vi "Initialize Logging Data.vi"(8 "error in (no error)":errorcluster, 11 "Device Ref in":T2=18446744073709551615 format="%.0x") -> (0 "error out":errorcluster, 1 "File Sample Specs":T9[](array[typedef]) {"File Status Ref" format="%.0x"; "Cmd Ref" format="%.0x"; "Data Loss Ref" format="%.0x"; "Error Ref" format="%.0x"; "Groups"."Decimation Ref" format="%.0x"; "Groups"."Block Refs"."Data Reference" format="%.0x"; "Trigger Ref" format="%.0x"}, 2 "File Log Specs":T3[](array[typedef]) {"File Node Ref" format="%.0x"}, 3 "Device Ref out":T2=18446744073709551615 format="%.0x", 4 "Max Group Size":i32, 5 "FIFO % Ref":T1 format="%.0x", 6 "Max # Channel Groups":i32)   [LabVIEW 2027, in "Embedded Data Logger Engine.lvlib"]
uses:
  Embedded Data Logger Engine.lvlib
  File Sampling Specification.ctl
  <vilib>/NI VeriStand/Custom Device API/Data Reference.ctl
  Group Sampling Specification.ctl
  <vilib>/NI VeriStand/Custom Device API/Block Data Reference.ctl
  File Logging Specification.ctl
  Group Logging Specification.ctl
  Group Buffer Data.ctl
  Property Specification.ctl
  <vilib>/NI VeriStand/Custom Device API/Custom Device Item Ref.ctl
  Shared/Segment Files By.ctl
  Logging State.ctl
  <vilib>/NI VeriStand/Custom Device API/Data Access Type.ctl
  Shared/Constants.vi
  <vilib>/NI VeriStand/Custom Device Tools/Custom Device Utility Library/NI VeriStand - Search for All Items by GUID.vi
  <vilib>/NI VeriStand/Custom Device Tools/Custom Device Utility Library/NI VeriStand - Search for Item by GUID.vi
  <vilib>/NI VeriStand/Custom Device Tools/Custom Device Utility Library/NI VeriStand - Search for Item by Property.vi
  <vilib>/NI VeriStand/Custom Device API/Get Item Property (String Array).vi
  <vilib>/NI VeriStand/Custom Device Tools/Custom Device Utility Library/Custom Device Utility Library.lvlib
  <vilib>/NI VeriStand/Custom Device API/Custom Device API.lvlib
  Shared/Embedded Data Logger Shared.lvlib
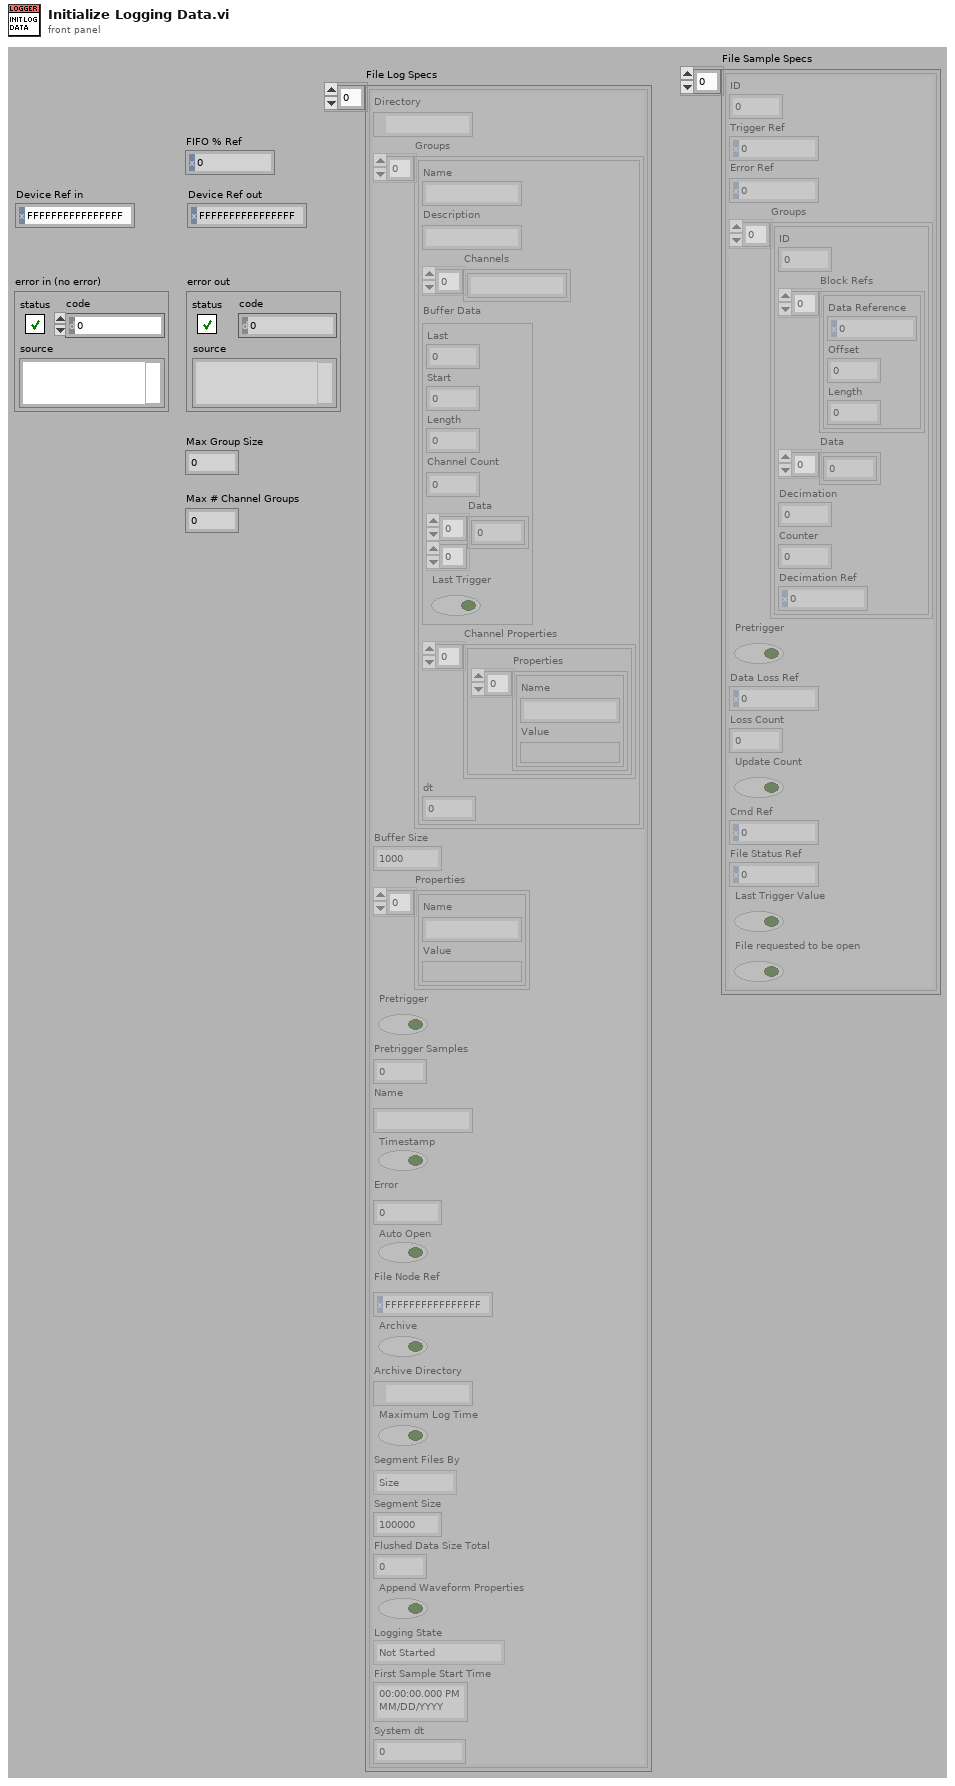
[diagram p1: front panel]
types:
  T1 = typedef "Custom Device API.lvlib/Data Reference.ctl" = i32
  T2 = typedef "Custom Device API.lvlib/Custom Device Item Ref.ctl" = u64
  T3 = typedef "Embedded Data Logger Engine.lvlib/File Logging Specification.ctl" = cluster{"Directory":path, "Groups":T4[], "Buffer Size":i32, "Properties":T6[], "Pretrigger":bool, "Pretrigger Samples":i32, "Name":string, "Timestamp":bool, "Error":i32, "Auto Open":bool, "File Node Ref":T2, "Archive":bool, "Archive Directory":path, "Segment Files":bool, "Segment Files By":T7, "Segment Size":u32, "Flushed Data Size Total":u32, "Append Waveform Properties":bool, "Logging State":T8, "First Sample Start Time":timestamp, "System dt":dbl}
  T4 = typedef "Embedded Data Logger Engine.lvlib/Group Logging Specification.ctl" = cluster{"Name":string, "Description":string, "Channels":string[], "Buffer Data":T5, "Channel Properties":cluster{"Properties":T6[]}[], "dt":dbl}
  T5 = typedef "Embedded Data Logger Engine.lvlib/Group Buffer Data.ctl" = cluster{"Last":i32, "Start":i32, "Length":i32, "Channel Count":i32, "Data":dbl[][], "Last Trigger":bool}
  T6 = typedef "Embedded Data Logger Engine.lvlib/Property Specification.ctl" = cluster{"Name":string, "Value":variant}
  T7 = typedef "Embedded Data Logger Shared.lvlib/Segment Files By.ctl" = enum16{"Time", "Size"}
  T8 = typedef "Embedded Data Logger Engine.lvlib/Logging State.ctl" = enum16{"Not Started", "Continous Logging", "Paused", "Discontinous Logging"}
  T9 = typedef "Embedded Data Logger Engine.lvlib/File Sampling Specification.ctl" = cluster{"ID":dbl, "Trigger Ref":T1, "Error Ref":T1, "Groups":T10[], "Pretrigger":bool, "Data Loss Ref":T1, "Loss Count":i32, "Update Count":bool, "Cmd Ref":T1, "File Status Ref":T1, "Last Trigger Value":bool, "File requested to be open":bool}
  T10 = typedef "Embedded Data Logger Engine.lvlib/Group Sampling Specification.ctl" = cluster{"ID":dbl, "Block Refs":T11[], "Data":dbl[], "Decimation":i32, "Counter":i32, "Decimation Ref":T1}
  T11 = typedef "Custom Device API.lvlib/Block Data Reference.ctl" = cluster{"Data Reference":T1, "Offset":u64, "Length":u64}
  T12 = typedef "Custom Device API.lvlib/Data Access Type.ctl" = enum16{"Read", "Write"}
  T13 = typedef "Custom Device API.lvlib/Custom Device Channel.ctl" = cluster{"Type":T14, "Units":string, "Default Value":dbl, "Faultable":bool, "Scalable":bool}
  T14 = typedef "Custom Device API.lvlib/Custom Device Channel Type.ctl" = enum16{"Input", "Output"}
  T15 = typedef "Custom Device API.lvlib/Custom Device Item Info.ctl" = cluster{"Name":string, "Is Channel":bool, "GUID":string, "Is Waveform":bool}
  T16 = cluster{cluster{"Name":string, "Variant":variant}[]}
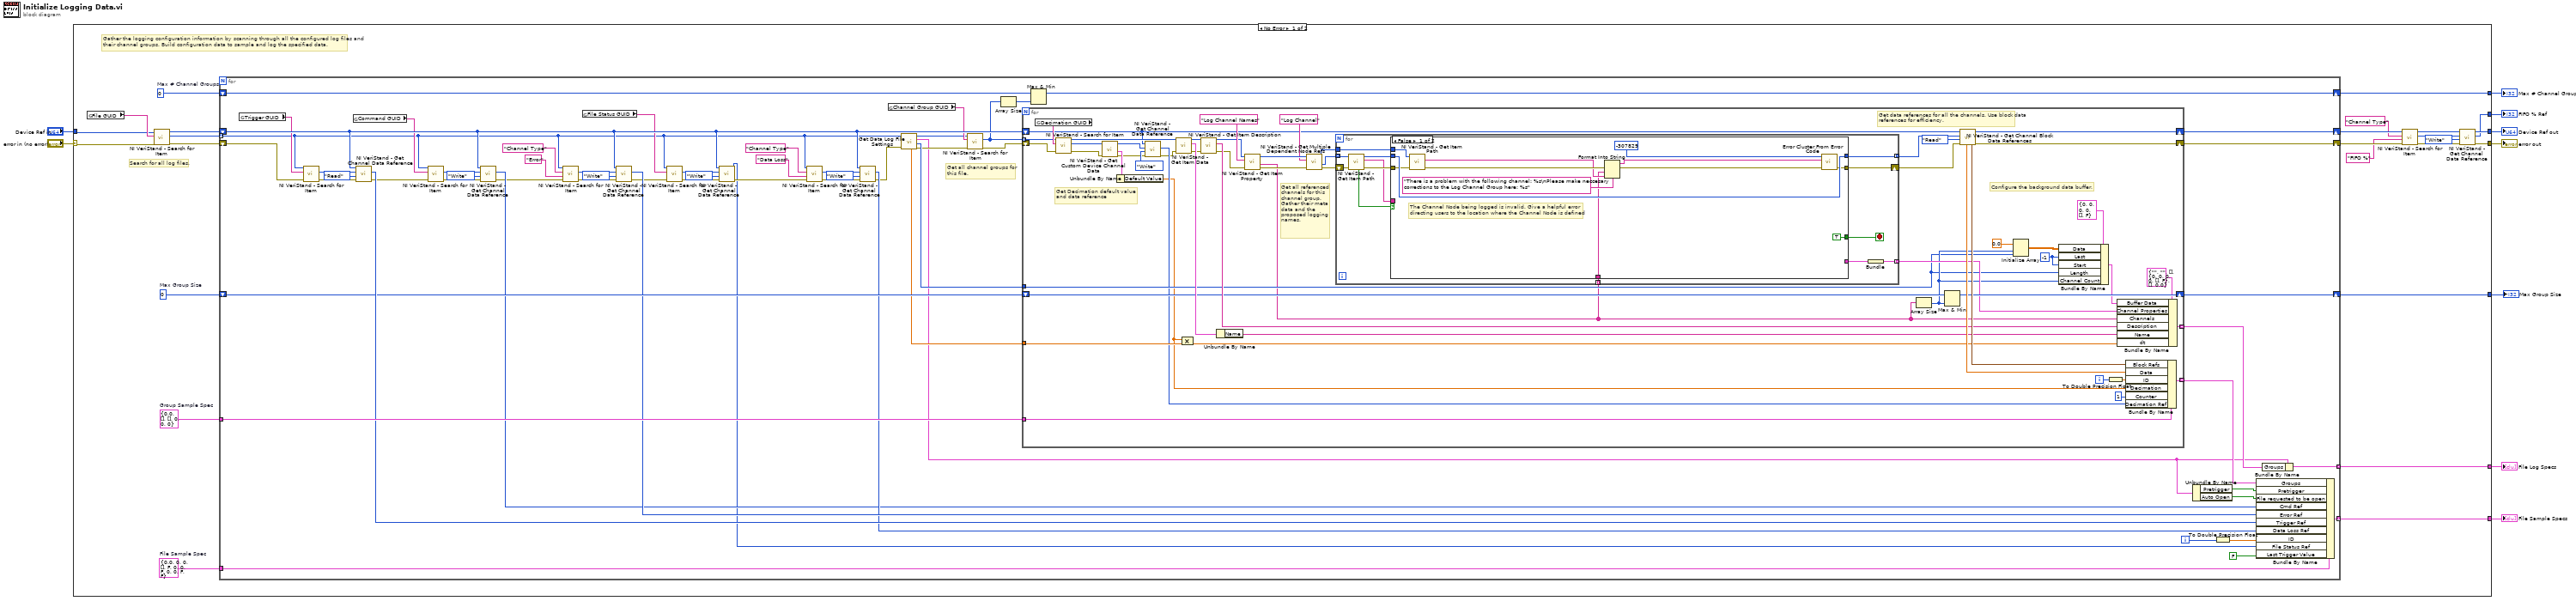
[diagram p0: block diagram]
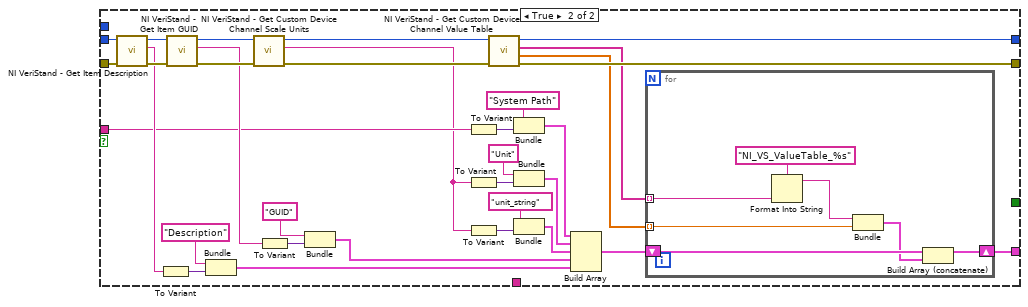
[diagram p2: hidden frame]
diagram:
  n1 = case shown="No Error" "error in (no error)" {
    selector: "error in (no error)" -> [w12 w217]
    tunnel: [w17 w217] -> w9
    tunnel: "Device Ref in" -> [w13 w216]
    tunnel: [w31 _] -> w6
    tunnel: [w20 w216] -> w5
    tunnel: [w28 _] -> w4
    tunnel: [w27 _] -> w3
    tunnel: [w15 _] -> w2
    tunnel: [w10 _] -> w1
    frame No Error {
      w11 = 0  # Max # Channel Groups
      w29 = T10 {"ID"=0.0, "Block Refs"=[], "Data"=[], "Decimation"=0, "Counter"=0, "Decimation Ref"=0}  # Group Sample Spec
      w32 = T9 {"ID"=0.0, "Trigger Ref"=0, "Error Ref"=0, "Groups"=[], "Pretrigger"=FALSE, "Data Loss Ref"=0, "Loss Count"=0, "Update Count"=FALSE, "Cmd Ref"=0, "File Status Ref"=0, "Last Trigger Value"=FALSE, "File requested to be open"=FALSE}  # File Sample Spec
      w26 = 0  # Max Group Size
      # "Search for all log files."
      # "Gather the logging configuration information by scanning through all the configured log files and their channel groups. Build configuration data to sample and log the specified data."
      n2 = global read "Constants.vi" "File GUID"() -> (w14:string)
      n3 = call-poly <vilib>:"NI VeriStand - Search for Item.vi"("error in"=w12, "Item GUID"=w14, "Section Ref in"=w13) -> ("error out"=w34:errorcluster, "Item Refs"=w33:T2[], "Section Ref out"=w30:T2)  [unwired: 1 in, 5 out]
      n4 = for {
        shift-right: [w85] -> w24
        shift-left: w34 -> [w52]
        tunnel: w33 -> [w47] mode=indexing
        tunnel: w32 -> [w95]
        tunnel: [w90] -> w31 mode=indexing
        shift-right: [w89] -> w25
        shift-left: w30 -> [w59]
        tunnel: w29 -> [w88]
        tunnel: [w83] -> w28 mode=indexing
        shift-right: [w38] -> w27
        shift-left: w26 -> [w81]
        shift-right: [w36] -> w10
        shift-left: w11 -> [w37]
        i -> [w94]
        # "Get all channel groups for\nthis file."
        n5 = global read "Constants.vi" "Trigger GUID"() -> (w56:string)
        n6 = call-poly <vilib>:"NI VeriStand - Search for Item.vi"("error in"=w52, "Item GUID"=w56, "Section Ref in"=w47) -> ("error out"=w86:errorcluster, "Item Ref"=w87:T2)  [unwired: 7 out]
        n7 = global read "Constants.vi" "Command GUID"() -> (w55:string)
        n8 = call <vilib>:"NI VeriStand - Get Channel Data Reference.vi"("error in (no error)"=w86, "Access"=Data_Access_Type."Read", "Channel Ref in"=w87, "Device Ref in"=w59) -> ("error out"=w65:errorcluster, "Channel Data Reference"=w84:T1)  [unwired: 6 out]
        n9 = call-poly <vilib>:"NI VeriStand - Search for Item.vi"("error in"=w65, "Item GUID"=w55, "Section Ref in"=w47) -> ("error out"=w67:errorcluster, "Item Ref"=w66:T2)  [unwired: 7 out]
        n10 = call <vilib>:"NI VeriStand - Get Channel Data Reference.vi"("error in (no error)"=w67, "Access"=Data_Access_Type."Write", "Channel Ref in"=w66, "Device Ref in"=w59) -> ("error out"=w49:errorcluster, "Channel Data Reference"=w64:T1)  [unwired: 6 out]
        n11 = call-poly <vilib>:"NI VeriStand - Search for Item.vi"("error in"=w49, "Property Value"="Error" ("Property Name"), "Property Name"="Channel Type", "Section Ref in"=w47) -> ("error out"=w79:errorcluster, "Item Ref"=w78:T2)  [unwired: 6 out]
        n12 = global read "Constants.vi" "File Status GUID"() -> (w54:string)
        n13 = call <vilib>:"NI VeriStand - Get Channel Data Reference.vi"("error in (no error)"=w79, "Access"=Data_Access_Type."Write", "Channel Ref in"=w78, "Device Ref in"=w59) -> ("error out"=w60:errorcluster, "Channel Data Reference"=w75:T1)  [unwired: 6 out]
        n14 = call-poly <vilib>:"NI VeriStand - Search for Item.vi"("error in"=w60, "Item GUID"=w54, "Section Ref in"=w47) -> ("error out"=w62:errorcluster, "Item Ref"=w63:T2)  [unwired: 7 out]
        n15 = call <vilib>:"NI VeriStand - Get Channel Data Reference.vi"("error in (no error)"=w62, "Access"=Data_Access_Type."Write", "Channel Ref in"=w63, "Device Ref in"=w59) -> ("error out"=w58:errorcluster, "Channel Data Reference"=w57:T1)  [unwired: 6 out]
        n16 = call-poly <vilib>:"NI VeriStand - Search for Item.vi"("error in"=w58, "Property Value"="Data Loss" ("Property Name"), "Property Name"="Channel Type", "Section Ref in"=w47) -> ("error out"=w71:errorcluster, "Item Ref"=w72:T2)  [unwired: 6 out]
        n17 = call <vilib>:"NI VeriStand - Get Channel Data Reference.vi"("error in (no error)"=w71, "Access"=Data_Access_Type."Write", "Channel Ref in"=w72, "Device Ref in"=w59) -> ("error out"=w48:errorcluster, "Channel Data Reference"=w69:T1)  [unwired: 6 out]
        n18 = global read "Constants.vi" "Channel Group GUID"() -> (w53:string)
        n19 = call "Get Data Log File Settings.vi"("error in"=w48, "File Ref in"=w47) -> ("error out"=w45:errorcluster, "Pretrigger Samples"=w50:i32, "File Log Specification"=w42:T3, "File Ref Out"=w46:T2, "System dt"=w51:dbl)  [unwired: 5 in]
        n20 = call-poly <vilib>:"NI VeriStand - Search for Item.vi"("error in"=w45, "Item GUID"=w53, "Section Ref in"=w46) -> ("error out"=w92:errorcluster, "Item Refs"=w40:T2[])  [unwired: 1 in, 6 out]
        n21 = Array Size(array=w40) -> (size(s)=w39:i32)
        n22 = for {
          shift-right: [w137] -> w85
          shift-left: w92 -> [w108]
          tunnel: w40 -> [w107] mode=indexing
          tunnel: [w148] -> w91 mode=indexing
          tunnel: w88 -> [w147]
          shift-right: [w134] -> w89
          shift-left: w59 -> [w105]
          tunnel: [w136] -> w43 mode=indexing
          shift-right: [w133] -> w38
          shift-left: w81 -> [w132]
          tunnel: w50 -> [w124]
          tunnel: w51 -> [w123]
          i -> [w145]
          w128 = -1 ("Last")
          # "Get Decimation default value and data reference"
          # "Get data references for all the channels. Use block data references for efficiency."
          # "Configure the background data buffer."
          # "Get all referenced channels for this channel group. Gather their meta data and the proposed logging names."
          n23 = global read "Constants.vi" "Decimation GUID"() -> (w109:string)
          n24 = call-poly <vilib>:"NI VeriStand - Search for Item.vi"("error in"=w108, "Item GUID"=w109, "Section Ref in"=w107) -> ("error out"=w98:errorcluster, "Item Ref"=w100:T2, "Section Ref out"=w106:T2)  [unwired: 6 out]
          n25 = call <vilib>:"NI VeriStand - Get Custom Device Channel Data.vi"("error in (no error)"=w98, "Channel Ref in"=w100) -> ("error out"=w97:errorcluster, "Channel"=w101:T13, "Channel Ref out"=w99:T2)  [unwired: 4 in, 3 out]
          n26 = Unbundle By Name(w101) -> ("Default Value"=w96:dbl)
          n27 = call <vilib>:"NI VeriStand - Get Channel Data Reference.vi"("error in (no error)"=w97, "Access"=Data_Access_Type."Write", "Channel Ref in"=w99, "Device Ref in"=w105) -> ("error out"=w103:errorcluster, "Channel Data Reference"=w104:T1)  [unwired: 6 out]
          n28 = call <vilib>:"NI VeriStand - Get Item Data.vi"("error in (no error)"=w103, "Item Ref in"=w106) -> ("error out"=w139:errorcluster, "Item Info"=w149:T15, "Item Ref out"=w140:T2)  [unwired: 7 out]
          n29 = Compound Arithmetic op=MULTIPLY(w96, w123) -> (w122:dbl)
          n30 = call <vilib>:"NI VeriStand - Get Item Description.vi"("error in (no error)"=w139, "Item Ref in"=w140) -> ("error out"=w118:errorcluster, "Description"=w138:string, "Item Ref out"=w119:T2)  [unwired: 7 out]
          n31 = Unbundle By Name(w149) -> ("Name"=w110:string)
          n32 = call-poly <vilib>:"NI VeriStand - Get Item Property.vi"("error in (no error)"=w118, "Property Name"="Log Channel Names", "Item Ref in"=w119) -> ("error out"=w116:errorcluster, "Value"=w111:string[], "Item Ref out"=w117:T2)  [unwired: 1 in, 5 out]
          n33 = call <vilib>:"NI VeriStand - Get Multiple Dependent Node Refs.vi"("error in (no error)"=w116, "Base Property Name"="Log Channel" ("Property Name"), "Item Ref in"=w117) -> ("error out"=w114:errorcluster, "Dependent Node Refs"=w113:T2[], "Item Ref out"=w112:T2)  [unwired: 6 in]
          n34 = for {
            shift-right: [w155] -> w142
            shift-left: w114 -> [w160]
            tunnel: [w156] -> w144 mode=indexing
            tunnel: [w162] -> w131 mode=indexing
            tunnel: w113 -> [w161] mode=indexing
            tunnel: w112 -> [w153]
            tunnel: w111 -> [w152] mode=indexing
            stop <- w151 stop-if-true
            n35 = call <vilib>:"NI VeriStand - Get Item Path.vi"("error in (no error)"=w160, "Item Ref in"=w161) -> ("error out"=w159:errorcluster, "Path"=w157:string, "Item Ref out"=w158:T2, "Found"=w154:bool)  [unwired: 6 in]
            n36 = case shown="False" w154 {
              tunnel: [_ w179] -> w163
              tunnel: w159 -> [w173 w190]
              tunnel: w158 -> [w175 w189]
              tunnel: w157 -> [_ w184]
              tunnel: [w175 w181] -> w156
              tunnel: [w167 w180] -> w155
              tunnel: w153 -> [w174 _]
              tunnel: w152 -> [w165 _]
              tunnel: [TRUE _] -> w151
              frame False {
                # "The Channel Node being logged is invalid. Give a helpful error \ndirecting users to the location where the Channel Node is defined"
                n37 = call <vilib>:"NI VeriStand - Get Item Path.vi"("error in (no error)"=w173, "Item Ref in"=w174) -> ("error out"=w168:errorcluster, "Path"=w166:string)  [unwired: 6 in, 2 out]
                n38 = Format Into String(format string="There is a problem with the following channel: %s\nPlease make neccesary corrections to the Log Channel Group here: %s" ("initial string"), error in=w168, w165, w166) -> (resulting string=w171:string, error out=w169:errorcluster)  [unwired: 1 in]
                n39 = call <vilib>:"Error Cluster From Error Code.vi"("error in (no error)"=w169, "error message (\"\")"=w171, "error code (0)"=-307829 ("Code")) -> ("error out"=w167:errorcluster)  [unwired: 6 in]
              }
              frame True {
                n40 = call <vilib>:"NI VeriStand - Get Item Description.vi"("error in (no error)"=w190, "Item Ref in"=w189) -> ("error out"=w205:errorcluster, "Description"=w204:string, "Item Ref out"=w206:T2)  [unwired: 7 out]
                n41 = To Variant(anything=w204) -> (Variant=w203:variant)
                n42 = call <vilib>:"NI VeriStand - Get Item GUID.vi"("error in (no error)"=w205, "Item Ref in"=w206) -> ("error out"=w207:errorcluster, "GUID"=w199:string, "Item Ref out"=w185:T2)  [unwired: 7 out]
                n43 = Bundle("Name"="Description", "Variant"=w203) -> (w197:cluster{"Name":string, "Variant":variant})  [unwired: 1 out]
                n44 = call <vilib>:"NI VeriStand - Get Custom Device Channel Scale Units.vi"("error in (no error)"=w207, "Channel Ref in"=w185) -> ("error out"=w208:errorcluster, "ScaleUnits"=w183:string, "Channel Ref out"=w182:T2)  [unwired: 7 in]
                n45 = To Variant(anything=w199) -> (Variant=w200:variant)
                n46 = Bundle("Name"="GUID", "Variant"=w200) -> (w198:cluster{"Name":string, "Variant":variant})  [unwired: 1 out]
                n47 = To Variant(anything=w184) -> (Variant=w192:variant)
                n48 = To Variant(anything=w183) -> (Variant=w196:variant)
                n49 = To Variant(anything=w183) -> (Variant=w187:variant)
                n50 = call <vilib>:"NI VeriStand - Get Custom Device Channel Value Table.vi"("error in (no error)"=w208, "Channel Ref in"=w182) -> ("error out"=w180:errorcluster, "Values"=w176:dbl[], "Names"=w177:string[], "Channel Ref out"=w181:T2)  [unwired: 6 in]
                n51 = Bundle("Name"="System Path", "Variant"=w192) -> (w191:cluster{"Name":string, "Variant":variant})  [unwired: 1 out]
                n52 = Bundle("Name"="Unit", "Variant"=w196) -> (w194:cluster{"Name":string, "Variant":variant})  [unwired: 1 out]
                n53 = Bundle("Name"="unit_string", "Variant"=w187) -> (w186:cluster{"Name":string, "Variant":variant})  [unwired: 1 out]
                n54 = Build Array(w191, w194, w186, w198, w197) -> (w178:cluster{"Name":string, "Variant":variant}[])
                n55 = for {
                  shift-right: [w214] -> w179
                  shift-left: w178 -> [w215]
                  tunnel: w177 -> [w211] mode=indexing
                  tunnel: w176 -> [w210] mode=indexing
                  n56 = Format Into String(format string="NI_VS_ValueTable_%s" ("Name"), w211) -> (resulting string=w212:string)  [unwired: 2 in, 1 out]
                  n57 = Bundle(w212, w210) -> (w209:cluster{string, dbl})  [unwired: 1 out]
                  n58 = Build Array (concatenate)(w215, w209) -> (w214:cluster{"Name":string, "Variant":variant}[])
                }
              }
            }
            n59 = Bundle(w163) -> (w162:T16)  [unwired: 1 in]
          }
          n60 = Array Size(array=w111) -> (size(s)=w125:i32)
          n61 = Max & Min(x=w132, y=w125) -> (max(x,y)=w133:i32)  [unwired: 1 out]
          n62 = call <vilib>:"NI VeriStand - Get Channel Block Data References.vi"("error in (no error)"=w142, "Access"=Data_Access_Type."Read", "Channel Refs"=w144, "Device Ref in"=w105) -> ("error out"=w137:errorcluster, "Values Array"=w150:dbl[], "Block Data Refs"=w141:T11[], "Device Ref out"=w134:T2)  [unwired: 4 out]
          n63 = Initialize Array(0.0 ("element"), w125, w124) -> (w126:dbl[][])
          n64 = Bundle By Name(cluster=T5 {"Last"=0, "Start"=0, "Length"=0, "Channel Count"=0, "Data"=[], "Last Trigger"=FALSE} ("Buffer Data"), "Data"=w126, "Last"=w128, "Start"=w128, "Length"=w124, "Channel Count"=w125) -> (w129:T5)
          n65 = To Double Precision Float(number=w145) -> (double precision float=w146:dbl)
          n66 = Bundle By Name(cluster=T4 {"Name"="", "Description"="", "Channels"=[], "Buffer Data"={"Last"=0, "Start"=0, "Length"=0, "Channel Count"=0, "Data"=[], "Last Trigger"=FALSE}, "Channel Properties"=[], "dt"=0.0} ("Group Log Spec"), "Buffer Data"=w129, "Channel Properties"=w131, "Channels"=w111, "Description"=w138, "Name"=w110, "dt"=w122) -> (w148:T4)
          n67 = Bundle By Name(cluster=w147, "Block Refs"=w141, "Data"=w150, "ID"=w146, "Decimation"=w96, "Counter"=1, "Decimation Ref"=w104) -> (w136:T10)
        }
        n68 = Max & Min(x=w37, y=w39) -> (max(x,y)=w36:i32)  [unwired: 1 out]
        n69 = Unbundle By Name(w42) -> ("Pretrigger"=w44:bool, "Auto Open"=w35:bool)
        n70 = To Double Precision Float(number=w94) -> (double precision float=w93:dbl)
        n71 = Bundle By Name(cluster=w95, "Groups"=w43, "Pretrigger"=w44, "File requested to be open"=w35, "Cmd Ref"=w64, "Error Ref"=w75, "Trigger Ref"=w84, "Data Loss Ref"=w69, "ID"=w93, "File Status Ref"=w57, "Last Trigger Value"=FALSE) -> (w83:T9)
        n72 = Bundle By Name(cluster=w42, "Groups"=w91) -> (w90:T3)
      }
      n73 = call-poly <vilib>:"NI VeriStand - Search for Item.vi"("error in"=w24, "Property Value"="FIFO %" ("String"), "Property Name"="Channel Type" ("String"), "Section Ref in"=w25) -> ("error out"=w18:errorcluster, "Item Ref"=w19:T2, "Section Ref out"=w21:T2)  [unwired: 4 in, 1 out]
      n74 = call <vilib>:"NI VeriStand - Get Channel Data Reference.vi"("error in (no error)"=w18, "Access"=Data_Access_Type."Write", "Channel Ref in"=w19, "Device Ref in"=w21) -> ("error out"=w17:errorcluster, "Channel Data Reference"=w15:T1, "Device Ref out"=w20:T2)  [unwired: 5 in]
    }
    frame Error {
    }
  }
  "error out" <- w9
  "File Sample Specs" <- w4
  "File Log Specs" <- w6
  "Device Ref out" <- w5
  "Max Group Size" <- w3
  "FIFO % Ref" <- w2
  "Max # Channel Groups" <- w1
